vi "2021 Advent puzzle 04 score calc.vi"(11 "Bingo Card":i16[][](array[numeric])) -> (3 "Score of this card":i64)   [LabVIEW 2021]
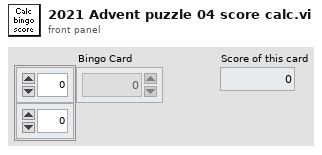
[diagram p1: front panel]
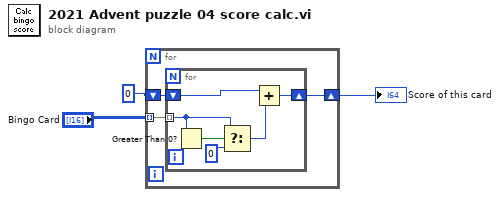
[diagram p0: block diagram]
diagram:
  n1 = for {
    tunnel: "Bingo Card" -> [w6] mode=indexing
    shift-right: [w4] -> w1
    shift-left: i64 0 ("Numeric 2") -> [w5]
    n2 = for {
      tunnel: w6 -> [w10] mode=indexing
      shift-right: [w7] -> w4
      shift-left: w5 -> [w12]
      n3 = Greater Than 0?(x=w10) -> (x > 0?=w11:bool)
      n4 = Select(t=w10, s=w11, f=i64 0) -> (s? t:f=w8:i64)
      n5 = Add(x=w12, y=w8) -> (x+y=w7:i64)
    }
  }
  "Score of this card" <- w1
